vi "Buttons.vi"() -> ()   [LabVIEW 2023]
panel:
  in  "stop":bool
  in  "Play Button 2":bool
  out "Boolean 2":bool
  in  "Play Button":bool
  out "Boolean":bool
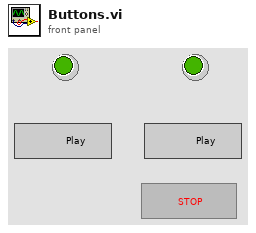
[diagram p1: front panel]
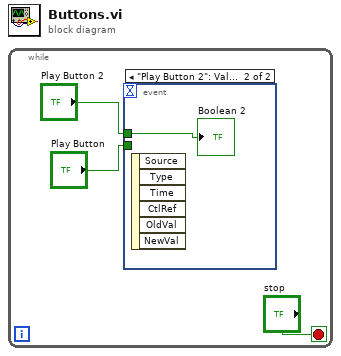
[diagram p0: block diagram]
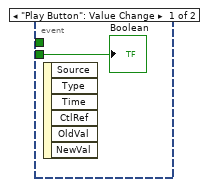
[diagram p2: hidden frame]
diagram:
  n1 = while {
    stop <- "stop" stop-if-true
    n2 = event shown="[1] \"Play Button 2\": Value Change" {
      selector: _ -> [_ _]
      dyn-events: _ -> [_ _]
      timeout: _ -> [_ _]
      tunnel: "Play Button" -> [w4 _]
      tunnel: "Play Button 2" -> [_ w5]
      event "Play Button": Value Change {
        n3 = event-data() -> ()  [unwired: 1 in, 6 out]
        "Boolean" <- w4
      }
      event "Play Button 2": Value Change {
        n4 = event-data() -> ()  [unwired: 1 in, 6 out]
        "Boolean 2" <- w5
      }
    }
  }
